vi "Examen_U1_V2.vi"() -> ()   [LabVIEW 2021]
uses:
  <vilib>/Instr/_visa.llb/VISA Configure Serial Port (Instr).vi
  <vilib>/express/express shared/transition.llb/Dynamic To Waveform Array.vi
  <vilib>/express/express signal manip/GetorSetDDTAttributes/Set DDT Attributes/SetT0.vi
  <vilib>/express/express shared/transition.llb/Waveform Array To Dynamic.vi
  <vilib>/express/express signal manip/GetorSetDDTAttributes/Set DDT Attributes/Set DDT Properties.xnode
panel:
  out "Dato Sensor\n LM-35":dbl
  in  "Terminar Lectura de Datos":bool
  in  "Terminar Ejecución del Programa":bool
  out "Temperatura actual":dbl
  out "Gráfica de Comportamiento":dynamicdata(graph)
  out "Tarjeta confirmada":bool
  out "Valor Mínimo":dbl
  out "Valor Máximo":dbl
  out "Indicador de la tarjeta":i32
  out "Tarjeta":string
  out "Lista de Tarjetas":string[](array[string])
  in  "Puerto de la Tarjeta":refnum<visa-resource-name>
  # "Instituto Politécnico Nacional"
  # "\"La técnica al servicio de la patria\"."
  # "Instrumentación Virtual Aplicada\nExamen U1"
  # "Gabriel Adame Cabrera\nDavid Irais García Valenzuela\nMaría Cristina Pérez Rico"
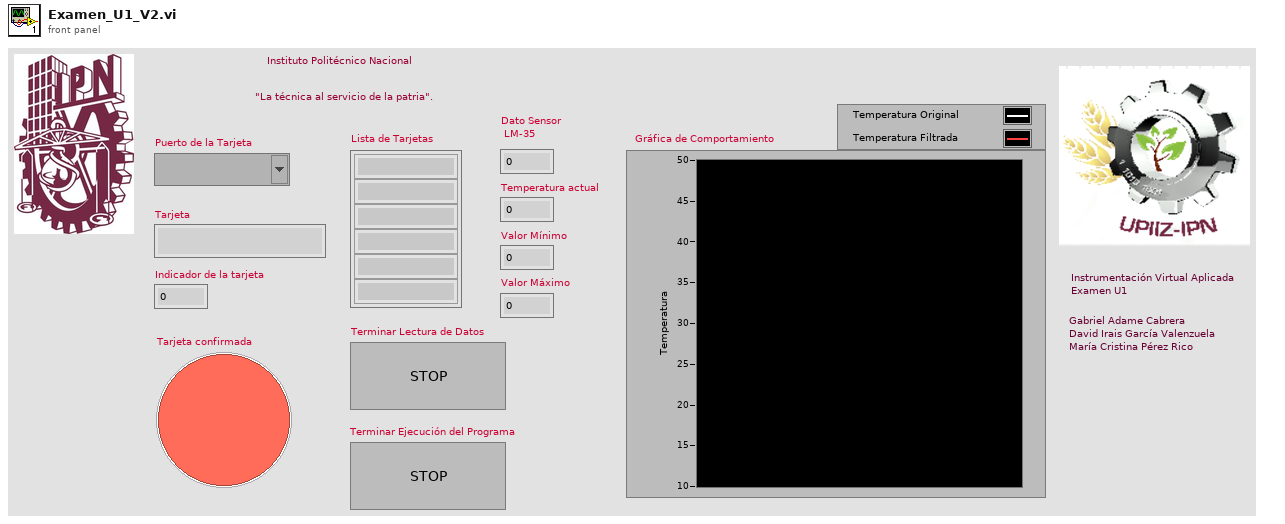
[diagram p1: front panel]
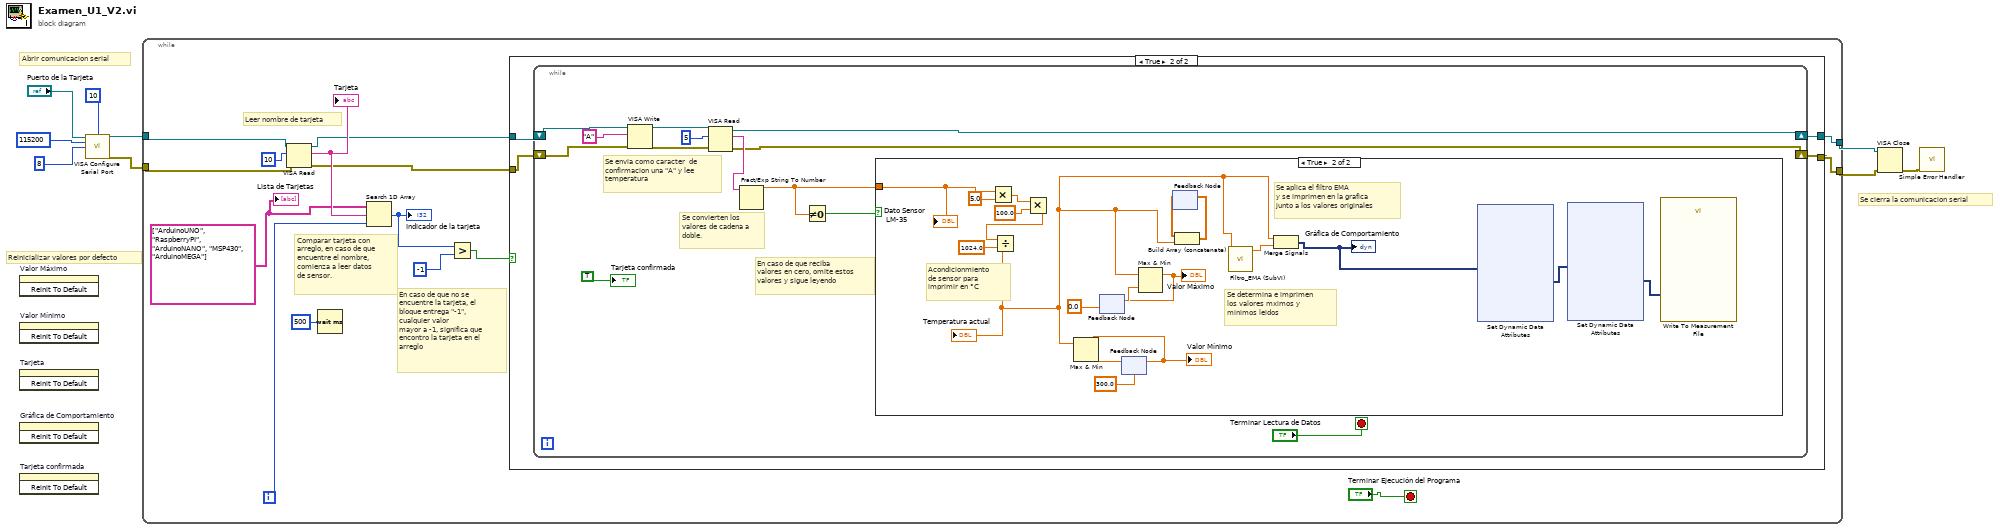
[diagram p0: block diagram]
diagram:
  # "Se cierra la comunicacion serial"
  # "Abrir comunicacion serial"
  # "Reinicializar valores por defecto"
  n1 = invoke on="Valor Máximo" class="DigNum (strict)" method="Reinit To Default"() -> ()  [unwired: 3 in, 3 out]
  n2 = invoke on="Valor Mínimo" class="DigNum (strict)" method="Reinit To Default"() -> ()  [unwired: 3 in, 3 out]
  n3 = invoke on="Tarjeta" class="Str" method="Reinit To Default"() -> ()  [unwired: 3 in, 3 out]
  n4 = invoke on="Gráfica de Comportamiento" class="WFChart (strict)" method="Reinit To Default"() -> ()  [unwired: 3 in, 3 out]
  n5 = invoke on="Tarjeta confirmada" class="Bool (strict)" method="Reinit To Default"() -> ()  [unwired: 3 in, 3 out]
  n6 = call-poly "VISA Configure Serial Port"("VISA resource name"="Puerto de la Tarjeta", "termination char\n(0xA = '\\n' = LF)"=u8 10 ("termination char\n(0xA = '\\n' = LF)"), "baud rate (9600)"=u32 115200, "data bits (8)"=u16 8) -> ("VISA resource name out"=w5:refnum<visa-resource-name>, "error out"=w6:errorcluster)  [unwired: 10 in]
  n7 = while {
    tunnel: w6 -> [w22]
    tunnel: w5 -> [w23]
    tunnel: [w14] -> w4
    tunnel: [w13] -> w3
    i -> [w21]
    stop <- "Terminar Ejecución del Programa" stop-if-true
    w10 = string[] ["ArduinoUNO", "RaspberryPI", "ArduinoNANO", "MSP430", "ArduinoMEGA"]
    # "En caso de que no se \nencuentre la tarjeta, el \nbloque entrega \"-1\", \ncualquier valor \nmayor a -1, significa que \nencontro la tarjeta en el\narreglo"
    # "Comparar tarjeta con \narreglo, en caso de que \nencuentre el nombre, \ncomienza a leer datos \nde sensor."
    # "Leer nombre de tarjeta"
    n8 = VISA Read(VISA resource name=w23, byte count=u32 10, error in (no error)=w22) -> (VISA resource name out=w16:refnum<visa-resource-name>, read buffer=w20:string, error out=w15:errorcluster)  [unwired: 1 out]
    "Tarjeta" <- w20
    n9 = Wait (ms)(milliseconds to wait=u32 500) -> ()  [unwired: 1 out]
    n10 = Search 1D Array(1D array=w10, element=w20, start index (0)=w21) -> (index of element=w19:i32)
    "Indicador de la tarjeta" <- w19
    n11 = Greater?(x=w19, y=-1) -> (0:w17:bool)
    n12 = case shown="True" w17 {
      tunnel: w16 -> [w26 w30]
      tunnel: w15 -> [w25 w29]
      tunnel: [w26 w28] -> w14
      tunnel: [w25 w27] -> w13
      frame False {
        # "En caso de que no encuentre la tarjeta en el arreglo, no se leen datos y la comunicacion se cierra."
      }
      frame True {
        n13 = while {
          shift-right: [w36] -> w28
          shift-left: w30 -> [w38]
          shift-right: [w35] -> w27
          shift-left: w29 -> [w37]
          stop <- "Terminar Lectura de Datos" stop-if-true
          # "Se convierten los \nvalores de cadena a\ndoble."
          # "En caso de que reciba \nvalores en cero, omite estos\nvalores y sigue leyendo"
          # "Se envia como caracter  de\nconfirmacion una \"A\" y lee \ntemperatura"
          n14 = VISA Write(VISA resource name=w38, write buffer="A", error in (no error)=w37) -> (VISA resource name out=w41:refnum<visa-resource-name>, error out=w40:errorcluster)  [unwired: 1 out]
          n15 = VISA Read(VISA resource name=w41, byte count=u32 5, error in (no error)=w40) -> (VISA resource name out=w36:refnum<visa-resource-name>, read buffer=w42:string, error out=w35:errorcluster)  [unwired: 1 out]
          n16 = Fract/Exp String To Number(string=w42) -> (number=w33:dbl)  [unwired: 3 in, 1 out]
          n17 = Not Equal To 0?(x=w33) -> (x != 0?=w32:bool)
          n18 = case shown="True" w32 {
            tunnel: w33 -> [_ w52]
            frame False {
              # "En caso de que se encuentre un cero, continua leyendo \ndatos y omite el cero."
            }
            frame True {
              # "Se determina e imprimen \nlos valores mximos y \nminimos leidos"
              # "Se aplica el filtro EMA \ny se imprimen en la grafica\njunto a los valores originales"
              # "Acondicionmiento \nde sensor para \nimprimir en °C"
              n19 = Multiply(x=w52, y=5.0) -> (x*y=w51:dbl)
              n20 = Multiply(x=w51, y=100.0) -> (x*y=w49:dbl)
              n21 = Divide(x=w49, y=1024.0) -> (x/y=w47:dbl)
              "Temperatura actual" <- w47
              n22 = feedback #1(0.0) -> (w61:dbl)
              n23 = feedback #2(300.0) -> (w58:dbl)
              n24 = Max & Min(x=w47, y=w58) -> (min(x,y)=w59:dbl)  [unwired: 1 out]
              "Valor Mínimo" <- w59
              n25 = feedback-in #2(w59) -> ()
              n26 = Max & Min(x=w47, y=w61) -> (max(x,y)=w60:dbl)  [unwired: 1 out]
              "Valor Máximo" <- w60
              n27 = feedback-in #1(w60) -> ()
              n28 = feedback #3() -> (w62:dbl[])  [unwired: 1 in]
              n29 = Build Array (concatenate)(w62, w47) -> (w55:dbl[])
              n30 = feedback-in #3(w55) -> ()
              n31 = call "Filtro_EMA (SubVI).vi"("Numeric in"=w47) -> ("Numeric out"=w54:dbl)  [unwired: 10 in]
              n32 = Merge Signals(w47, w54) -> (w46:dynamicdata)
              "Gráfica de Comportamiento" <- w46
              n33 = xnode "Set Dynamic Data Attributes"("Signals In"=w46) -> ("Signals Out"=w45:dynamicdata)  [unwired: 3 in, 1 out]
              n34 = xnode "Set Dynamic Data Attributes"("Signals In"=w45) -> ("Signals Out"=w44:dynamicdata)  [unwired: 3 in, 1 out]
              n35 = call "Write To Measurement File"("Signals"=w44) -> ()  [unwired: 16 in, 3 out]
              "Dato Sensor\n LM-35" <- w52
            }
          }
          "Tarjeta confirmada" <- TRUE ("Tarjeta confirmada")
        }
      }
    }
    "Lista de Tarjetas" <- w10
  }
  n36 = VISA Close(VISA resource name=w4, error in (no error)=w3) -> (error out=w1:errorcluster)
  n37 = call <vilib>:"Simple Error Handler.vi"("error in (no error)"=w1) -> ()  [unwired: 4 in, 5 out]
